vi "Pop.vi"(8 "error in (no error)":errorcluster, 11 "Stack in":refnum<class "Stack.lvclass">) -> (0 "error out":errorcluster, 2 "Element":dbl, 3 "Stack out":refnum<class "Stack.lvclass">)   [LabVIEW 2016, in "Stack.lvlib" / "Stack.lvclass"]
doc: "Pop an element from top of stack."
uses:
  Stack.lvclass
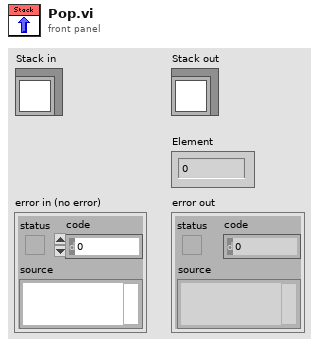
[diagram p1: front panel]
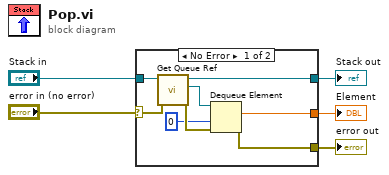
[diagram p0: block diagram]
diagram:
  n1 = case shown="No Error" "error in (no error)" {
    selector: "error in (no error)" -> [w9 w15]
    tunnel: [w8 w15] -> w4
    tunnel: [w12 w14] -> w2
    tunnel: "Stack in" -> [w13 w14]
    tunnel: [w7 _] -> w1
    frame No Error {
      n2 = call "Get Queue Ref.vi"("error in (no error)"=w9, "Stack in"=w13) -> ("error out"=w10:errorcluster, "queue out"=w11:refnum<queue>, "Stack out"=w12:refnum<class "Stack.lvclass">)  [unwired: 7 in]
      n3 = Dequeue Element(queue=w11, timeout in ms (-1)=0, error in (no error)=w10) -> (element=w7:dbl, error out=w8:errorcluster)  [unwired: 2 out]
    }
    frame Error {
    }
  }
  "error out" <- w4
  "Stack out" <- w2
  "Element" <- w1
